vi "Shooter2 Controller.vi"(8 "error in":errorcluster) -> ()   [LabVIEW 2019]
doc: "This VI executes continuously carrying out the current operation and responding to updates or new operations. It will often contain the timing or control code that is difficult to place directly in TeleOp. This VI generally opens all sensors and motors and isolates the rest of the robot code from knowing how the operations are carried out."
uses:
  Shooter2 Setpoints.ctl
  Shooter2 Operations.ctl
  <vilib>/Rock Robotics/WPI/ThirdParty/Phoenix-LabVIEW/Motor Controller/Controls/CTRE_Phoenix_MotorControl_FeedbackDevice.ctl
  <vilib>/Rock Robotics/WPI/ThirdParty/Phoenix-LabVIEW/Motor Controller/Controls/CTRE_Phoenix_MotorControl_NeutralMode.ctl
  <vilib>/Rock Robotics/WPI/ThirdParty/Phoenix-LabVIEW/Motor Controller/Controls/CTRE_Phoenix_MotorControl_ControlMode.ctl
  <vilib>/Rock Robotics/WPI/ThirdParty/Phoenix-LabVIEW/Motor Controller/Get/CTRE_Phoenix_MotorController_GetSelectedSensorData.vi
  <vilib>/Rock Robotics/Network Tables/NT Write Boolean.vi
panel:
  out "Current\nCmd":string
  # "Tip: It may be helpful to observe inputs and sensor values.\nYou may also want to display tuning or debugging controls."
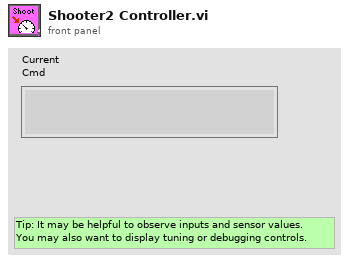
[diagram p1: front panel]
types:
  T1 = typedef "CTRE_Phoenix_MotorControl_ControlMode.ctl" = u16
  T2 = typedef "CTRE_Phoenix_MotorControl_NeutralMode.ctl" = enum8{"EEPROMSetting", "Override to Coast", "Override to Brake"}
  T3 = typedef "CTRE_Phoenix_MotorControl_FeedbackDevice.ctl" = i8
  T4 = typedef "Shooter2 Setpoints.ctl" = cluster{"Operation":T5, "Setpoint":dbl, "Duration":dbl}
  T5 = typedef "Shooter2 Operations.ctl" = enum16{"Reserve", "Read Current", "Immediate", "Shoot Manual", "Shoot Auto"}
  T6 = typedef "WPI_MotorControlDeviceRef.ctl" = cluster{"DeviceStatus":errorcluster, "Type":T7, "PWM":cluster{"PWM Channel":T8, "DeadBand":T9}, "CAN":cluster{"Device Number":u8, "SetOutput VI Ref":variant, "GetOutput VI Ref":variant, "Enable VI Ref":variant, "Disable VI Ref":variant, "Data":variant}, "Invert":bool, "DIO PWM":cluster{"PWM \"Enable\" Channel":T8, "DIOChannel":T10, "PWM Rate":dbl}}
  T7 = typedef "WPI_MotorControlType.ctl" = enum16{"PWM", "CAN", "DIO PWM"}
  T8 = typedef "FPGA_DIOPWMChannel.ctl" = enum8{"PWM 0", "PWM 1", "PWM 2", "PWM 3", "PWM 4", "PWM 5", "PWM 6", "PWM 7", "PWM 8", "PWM 9", "PWM MXP 0", "PWM MXP 1", "PWM MXP 2", "PWM MXP 3", "PWM MXP 4", "PWM MXP 5", "PWM MXP 6", "PWM MXP 7", "PWM MXP 8", "PWM MXP 9", "Invalid"}
  T9 = typedef "WPI_PWMDeadband.ctl" = cluster{"Name":string, "maxPositivePwm":i32, "minPositivePwm":i32, "centerPwm":i32, "maxNegativePwm":i32, "minNegativePwm":i32, "angularRange":u16}
  T10 = typedef "FPGA_DIOChannel.ctl" = enum8{"DIO 0", "DIO 1", "DIO 2", "DIO 3", "DIO 4", "DIO 5", "DIO 6", "DIO 7", "DIO 8", "DIO 9", "DIO MXP 0", "DIO MXP 1", "DIO MXP 2", "DIO MXP 3", "DIO MXP 4", "DIO MXP 5", "DIO MXP 6", "DIO MXP 7", "DIO MXP 8", "DIO MXP 9", "DIO MXP 10", "DIO MXP 11", "DIO MXP 12", "DIO MXP 13", "DIO MXP 14", "DIO MXP 15", "SPI Port CS1", "SPI Port CS2", "SPI Port CS3", "SPI Port MISO", "SPI Port MOSI", "Invalid"}
  T11 = typedef "Command Status Info.ctl" = cluster{"Name":string, "Status":T12, "notifier out":T13}
  T12 = typedef "Completion Status.ctl" = enum16{"Successful", "Aborted", "Incomplete"}
  T13 = typedef "Completion Notifier.ctl" = refnum<notifier>
  T14 = cluster{"Current Command":T4, "Command Timing":cluster{"Start Time (ms)":u32, "Iterations":i32}, "Command Arguments":cluster{"Command Info":T11, "Description":string, "Default Command":T4, "queue out":refnum<queue>, "Subsystem Name":string}}
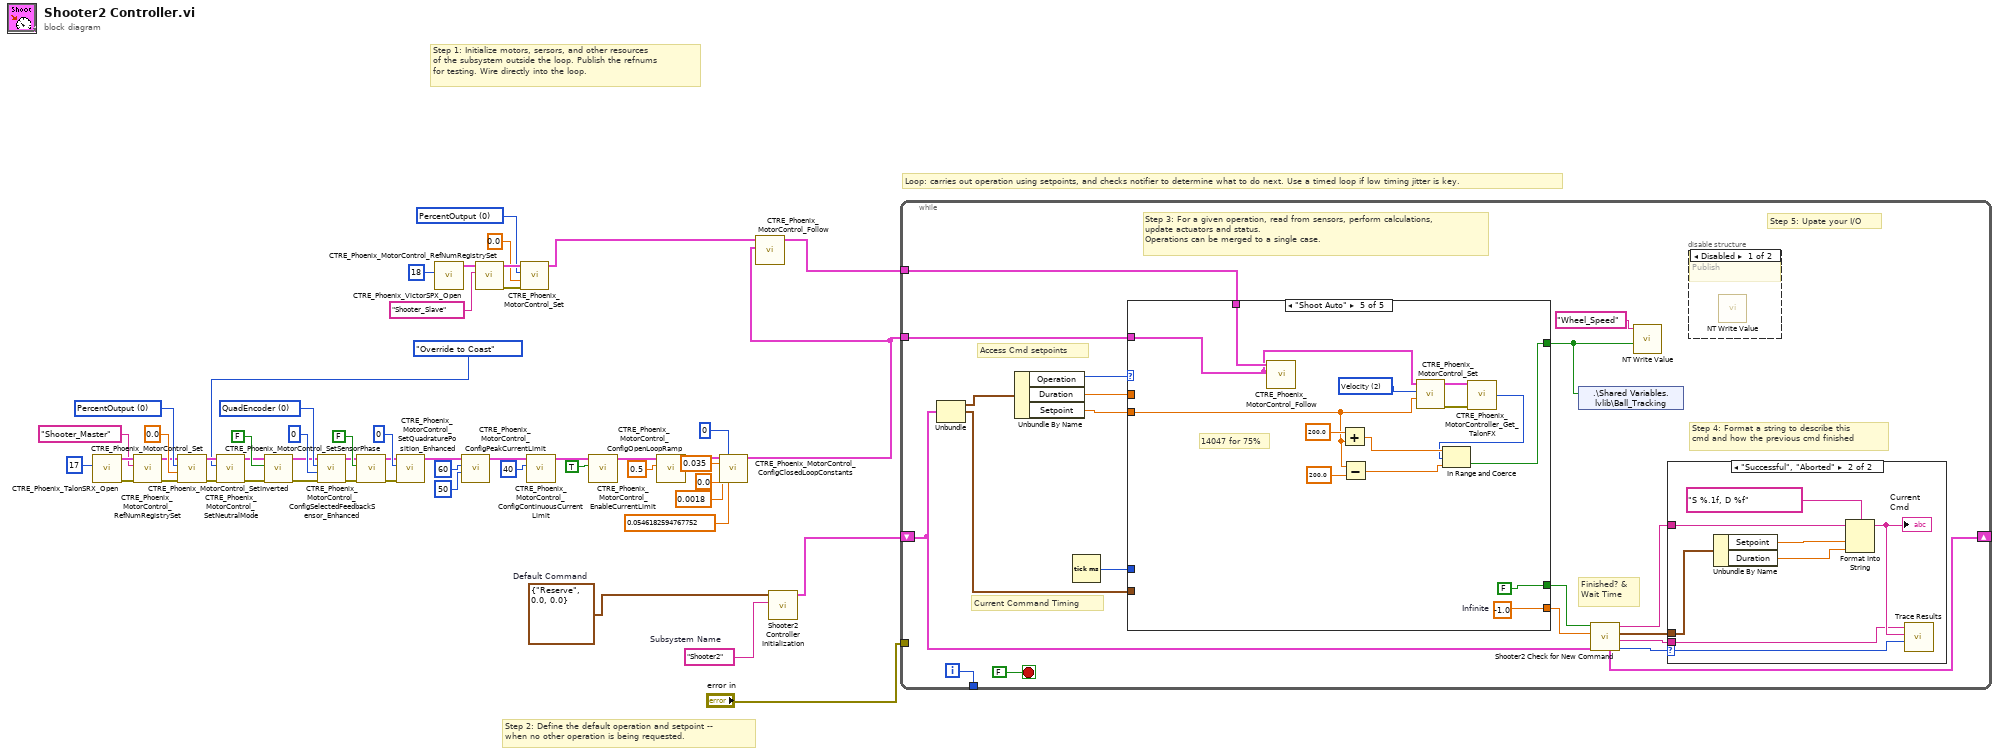
[diagram p0: block diagram]
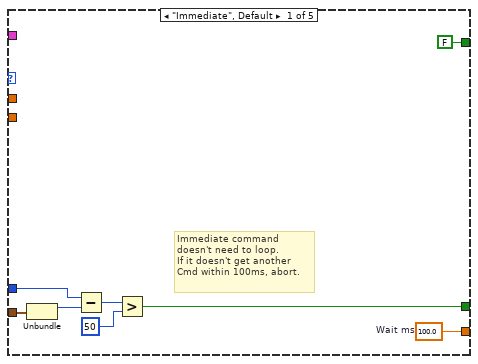
[diagram p4: hidden frame]
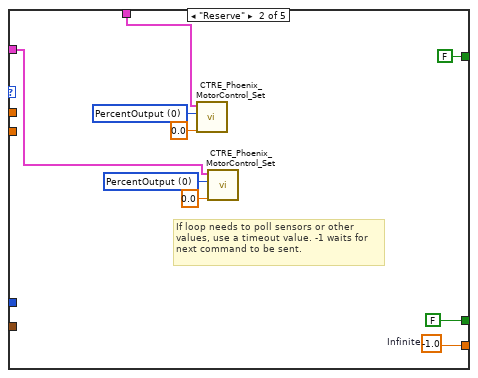
[diagram p5: hidden frame]
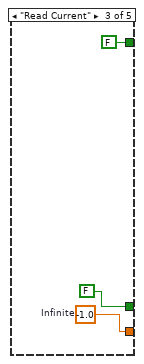
[diagram p6: hidden frame]
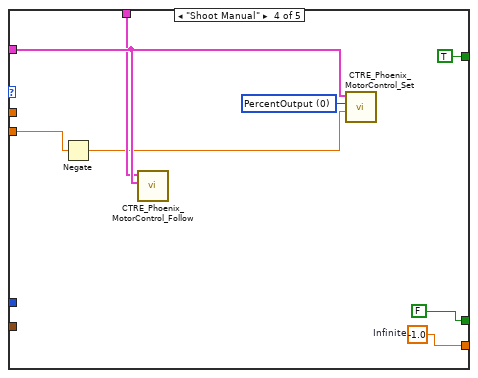
[diagram p7: hidden frame]
diagram:
  w19 = T1 0 items=["PercentOutput"=0, "Position"=1, "Velocity"=2, "Current"=3, "Follower"=5, "MotionProfile"=6, "MotionMagic"=7, "MotionProfileArc"=10, "Disabled"=15] ("Control Mode")
  w33 = T1 0 items=["PercentOutput"=0, "Position"=1, "Velocity"=2, "Current"=3, "Follower"=5, "MotionProfile"=6, "MotionMagic"=7, "MotionProfileArc"=10, "Disabled"=15] ("Control Mode")
  w46 = T3 0 items=["QuadEncoder"=0, "Analog"=2, "Tachometer"=4, "Pulse Width Encoded Position"=8, "Sensor Sum (S0 + S1)"=9, "Sensor Difference (D0 - D1)"=10, "Remote Source 0"=11, "Remote Source 1"=12, "Software Emulated"=15] ("Feedback Device")
  w49 = T4 {"Operation"=enum."Reserve", "Setpoint"=0.0, "Duration"=0.0}  # Default Command
  w50 = "Shooter2"  # Subsystem Name
  # "Step 2: Define the default operation and setpoint --\nwhen no other operation is being requested."
  # "Step 1: Initialize motors, sersors, and other resources\nof the subsystem outside the loop. Publish the refnums\nfor testing. Wire directly into the loop."
  # "Loop: carries out operation using setpoints, and checks notifier to determine what to do next. Use a timed loop if low timing jitter is key."
  n1 = call <vilib>:"CTRE_Phoenix_TalonSRX_Open.vi"("Device Number"=u8 17) -> ("error out"=w48:errorcluster, "CAN Talon SRX Ref"=w47:T6)  [unwired: 9 in]
  n2 = call <vilib>:"CTRE_Phoenix_MotorControl_RefNumRegistrySet.vi"("error in (no error)"=w48, "refnum name"="Shooter_Master", "PhoenixMotorControlDevRef"=w47) -> ("error out"=w30:errorcluster, "PhoenixMotorControlDevRef"=w31:T6)  [unwired: 7 in]
  n3 = call <vilib>:"CTRE_Phoenix_MotorControl_Set.vi"("error in (no error)"=w30, "Output"=0.0, "Control Mode"=w33, "PhoenixMotorControlDevRef"=w31) -> ("error out"=w29:errorcluster, "PhoenixMotorControlDevRef"=w35:T6)  [unwired: 6 in]
  n4 = call <vilib>:"CTRE_Phoenix_MotorControl_SetNeutralMode.vi"("error in (no error)"=w29, "Motor Control Neutral Mode"=CTRE_Phoenix_MotorControl_NeutralMode."Override to Coast", "PhoenixMotorControlDevRef"=w35) -> ("error out"=w28:errorcluster, "PhoenixMotorControlDevRef"=w36:T6)  [unwired: 7 in]
  n5 = call <vilib>:"CTRE_Phoenix_MotorControl_SetInverted.vi"("error in (no error)"=w28, "Invert?"=FALSE, "PhoenixMotorControlDevRef"=w36) -> ("error out"=w27:errorcluster, "PhoenixMotorControlDevRef"=w37:T6)  [unwired: 7 in]
  n6 = call <vilib>:"CTRE_Phoenix_MotorControl_ConfigSelectedFeedbackSensor_Enhanced.vi"("error in (no error)"=w27, "pidLoopIdx"=0, "Feedback Device"=w46, "PhoenixMotorControlDevRef"=w37) -> ("error out"=w39:errorcluster, "PhoenixMotorControlDevRef"=w41:T6)  [unwired: 6 in]
  n7 = call <vilib>:"CTRE_Phoenix_MotorControl_SetSensorPhase.vi"("error in (no error)"=w39, "PhaseSensor"=FALSE, "PhoenixMotorControlDevRef"=w41) -> ("error out"=w40:errorcluster, "PhoenixMotorControlDevRef"=w42:T6)  [unwired: 7 in]
  n8 = call <vilib>:"CTRE_Phoenix_MotorControl_SetQuadraturePosition_Enhanced.vi"("error in (no error)"=w40, "New Position"=0, "PhoenixMotorControlDevRef"=w42) -> ("PhoenixMotorControlDevRef"=w11:T6)  [unwired: 7 in, 1 out]
  n9 = call <vilib>:"CTRE_Phoenix_VictorSPX_Open.vi"("Device Number"=u8 18) -> ("CAN Talon SRX Ref"=w22:T6)  [unwired: 9 in, 1 out]
  n10 = call <vilib>:"CTRE_Phoenix_MotorControl_ConfigPeakCurrentLimit.vi"("Peak Current Maximum Duration (ms)"=50, "Peak Current (Amps)"=60, "PhoenixMotorControlDevRef"=w11) -> ("PhoenixMotorControlDevRef"=w13:T6)  [unwired: 7 in, 1 out]
  n11 = call <vilib>:"CTRE_Phoenix_MotorControl_RefNumRegistrySet.vi"("refnum name"="Shooter_Slave", "PhoenixMotorControlDevRef"=w22) -> ("error out"=w24:errorcluster, "PhoenixMotorControlDevRef"=w23:T6)  [unwired: 8 in]
  n12 = call <vilib>:"CTRE_Phoenix_MotorControl_Set.vi"("error in (no error)"=w24, "Output"=0.0, "Control Mode"=w19, "PhoenixMotorControlDevRef"=w23) -> ("PhoenixMotorControlDevRef"=w17:T6)  [unwired: 6 in, 1 out]
  n13 = call <vilib>:"CTRE_Phoenix_MotorControl_ConfigContinuousCurrentLimit.vi"("Continuous Current Limit (Amps)"=40, "PhoenixMotorControlDevRef"=w13) -> ("PhoenixMotorControlDevRef"=w12:T6)  [unwired: 8 in, 1 out]
  n14 = call <vilib>:"CTRE_Phoenix_MotorControl_EnableCurrentLimit.vi"("Enable Current Limit?"=TRUE, "PhoenixMotorControlDevRef"=w12) -> ("PhoenixMotorControlDevRef"=w8:T6)  [unwired: 8 in, 1 out]
  n15 = call <vilib>:"CTRE_Phoenix_MotorControl_ConfigOpenLoopRamp.vi"("secondsFromNeutralToFull"=0.5, "PhoenixMotorControlDevRef"=w8) -> ("PhoenixMotorControlDevRef"=w7:T6)  [unwired: 8 in, 1 out]
  n16 = call <vilib>:"CTRE_Phoenix_MotorControl_ConfigClosedLoopConstants.vi"("PhoenixMotorControlDevRef"=w7, "slotIdx"=0, "P"=0.035, "I"=0.0, "D"=0.0018, "F"=0.0546182594767752) -> ("PhoenixMotorControlDevRef"=w1:T6)  [unwired: 8 in, 1 out]
  n17 = call <vilib>:"CTRE_Phoenix_MotorControl_Follow.vi"("Master Controller to Follow"=w1, "PhoenixMotorControlDevRef"=w17) -> ()  [unwired: 8 in, 2 out]
  n18 = call "Shooter2 Controller Initialization.vi"("Subsystem Name"=w50, "Default Command"=w49) -> ("Current Command"=w51:T14)  [unwired: 9 in]
  n19 = while {
    shift-right: [w64] -> _
    shift-left: w51 -> [w57]
    tunnel: [w71] -> _
    tunnel: "error in" -> [_]
    tunnel: w1 -> [w56]
    tunnel: w17 -> [w55]
    i -> [w71]
    stop <- FALSE stop-if-true
    # "Step 5: Upate your I/O"
    # "Step 4: Format a string to describe this\ncmd and how the previous cmd finished"
    # "Current Command Timing"
    # "Access Cmd setpoints"
    # "Finished? &\nWait Time"
    # "Step 3: For a given operation, read from sensors, perform calculations,\nupdate actuators and status.\nOperations can be merged to a single case."
    n20 = Unbundle(w57) -> ("Current Command"=w70:T4, "Command Timing"=w66:cluster{"Start Time (ms)":u32, "Iterations":i32})  [unwired: 1 out]
    n21 = Unbundle By Name(w70) -> ("Operation"=w69:T5, "Duration"=w68:dbl, "Setpoint"=w65:dbl)
    n22 = Tick Count (ms)() -> (millisecond timer value=w67:u32)
    n23 = case shown="\"Shoot Auto\"" w69 {
      tunnel: [w88 w97 w99 w107 w122] -> w62
      tunnel: [w82 FALSE ("ignore previous (F)") FALSE ("ignore previous (F)") FALSE ("ignore previous (F)") FALSE ("ignore previous (F)")] -> w63
      tunnel: w66 -> [w84 _ _ _ _]
      tunnel: w68 -> [_ _ _ _ _]
      tunnel: w67 -> [w83 _ _ _ _]
      tunnel: w65 -> [_ _ _ w103 w111]
      tunnel: w56 -> [_ w91 _ w105 w118]
      tunnel: w55 -> [_ w90 _ w104 w119]
      tunnel: [FALSE FALSE FALSE TRUE w109] -> w53
      frame "Immediate", Default {
        w88 = 100.0  # Wait ms
        # "Immediate command\ndoesn't need to loop.\nIf it doesn't get another\nCmd within 100ms, abort."
        n24 = Unbundle(w84) -> ("Start Time (ms)"=w87:u32)  [unwired: 1 out]
        n25 = Subtract(x=w83, y=w87) -> (x-y=w86:u32)
        n26 = Greater?(x=w86, y=u8 50 ("Left Motor")) -> (0:w82:bool)
      }
      frame "Reserve" {
        w93 = T1 0 items=["PercentOutput"=0, "Position"=1, "Velocity"=2, "Current"=3, "Follower"=5, "MotionProfile"=6, "MotionMagic"=7, "MotionProfileArc"=10, "Disabled"=15] ("Control Mode")
        w95 = T1 0 items=["PercentOutput"=0, "Position"=1, "Velocity"=2, "Current"=3, "Follower"=5, "MotionProfile"=6, "MotionMagic"=7, "MotionProfileArc"=10, "Disabled"=15] ("Control Mode")
        w97 = -1.0  # Infinite
        # "If loop needs to poll sensors or other\nvalues, use a timeout value. -1 waits for\nnext command to be sent."
        n27 = call <vilib>:"CTRE_Phoenix_MotorControl_Set.vi"("Output"=0.0, "Control Mode"=w95, "PhoenixMotorControlDevRef"=w90) -> ()  [unwired: 7 in, 2 out]
        n28 = call <vilib>:"CTRE_Phoenix_MotorControl_Set.vi"("Output"=0.0, "Control Mode"=w93, "PhoenixMotorControlDevRef"=w91) -> ()  [unwired: 7 in, 2 out]
      }
      frame "Read Current" {
        w99 = -1.0  # Infinite
      }
      frame "Shoot Manual" {
        w106 = T1 0 items=["PercentOutput"=0, "Position"=1, "Velocity"=2, "Current"=3, "Follower"=5, "MotionProfile"=6, "MotionMagic"=7, "MotionProfileArc"=10, "Disabled"=15] ("Control Mode")
        w107 = -1.0  # Infinite
        n29 = Negate(x=w103) -> (-x=w102:dbl)
        n30 = call <vilib>:"CTRE_Phoenix_MotorControl_Follow.vi"("Master Controller to Follow"=w105, "PhoenixMotorControlDevRef"=w104) -> ()  [unwired: 8 in, 2 out]
        n31 = call <vilib>:"CTRE_Phoenix_MotorControl_Set.vi"("Output"=w102, "Control Mode"=w106, "PhoenixMotorControlDevRef"=w105) -> ()  [unwired: 7 in, 2 out]
      }
      frame "Shoot Auto" {
        w120 = T1 2 items=["PercentOutput"=0, "Position"=1, "Velocity"=2, "Current"=3, "Follower"=5, "MotionProfile"=6, "MotionMagic"=7, "MotionProfileArc"=10, "Disabled"=15] ("Control Mode")
        w122 = -1.0  # Infinite
        # "14047 for 75%"
        n32 = call <vilib>:"CTRE_Phoenix_MotorControl_Follow.vi"("Master Controller to Follow"=w118, "PhoenixMotorControlDevRef"=w119) -> ()  [unwired: 8 in, 2 out]
        n33 = Add(x=200.0, y=w111) -> (x+y=w114:dbl)
        n34 = Subtract(x=w111, y=200.0) -> (x-y=w115:dbl)
        n35 = call <vilib>:"CTRE_Phoenix_MotorControl_Set.vi"("Output"=w111, "Control Mode"=w120, "PhoenixMotorControlDevRef"=w118) -> ("error out"=w116:errorcluster, "PhoenixMotorControlDevRef"=w117:T6)  [unwired: 7 in]
        n36 = call-poly <vilib>:"CTRE_Phoenix_MotorController_Get_TalonFX.vi"("PhoenixMotorControlDevRef"=w117, "error in"=w116) -> ("Velocity (Raw Sensor Units per 100 ms)"=w110:i32)  [unwired: 10 in, 3 out]
        n37 = In Range and Coerce(upper limit=w114, x=w110, lower limit=w115) -> (In Range?=w109:bool)  [unwired: 1 out]
      }
    }
    n38 = shared-variable ".\\Shared Variables.lvlib\\Ball_Tracking"(w53) -> ()  [unwired: 1 in, 1 out]
    n39 = call "Shooter2 Check for New Command.vi"("Current Command"=w57, "Wait time (ms)"=w62, "Finished?"=w63) -> ("Completion"=w58:T12, "Subsystem Name"=w59:string, "Current Command"=w60:T4, "Initial Trace String"=w61:string, "NextCommand"=w64:T14)  [unwired: 4 in]
    n40 = call-poly <vilib>:"NT Write Value.vi"("Boolean"=w53, "Name"="Wheel_Speed") -> ()  [unwired: 9 in, 1 out]
    n41 = case shown="\"Successful\", \"Aborted\"" w58 {
      selector: w58 -> [_ w80]
      tunnel: w61 -> [_ w76]
      tunnel: w60 -> [_ w77]
      tunnel: w59 -> [_ w73]
      frame "Incomplete", Default {
        # "Continuing current command"
      }
      frame "Successful", "Aborted" {
        # "Report and setup for next command"
        n42 = Unbundle By Name(w77) -> ("Setpoint"=w79:dbl, "Duration"=w74:dbl)
        n43 = Format Into String(format string="S %.1f, D %f", initial string=w76, w79, w74) -> (resulting string=w75:string)  [unwired: 1 in, 1 out]
        "Current\nCmd" <- w75
        n44 = call <vilib>:"Trace Results.vi"("Status of previous command"=w80, "Description"=w75, "Subsystem"=w73) -> ()  [unwired: 9 in]
      }
    }
    n45 = disable-structure shown="Disabled" {
      frame Disabled {
        # "Publish"
        n46 = call-poly <vilib>:"NT Write Value.vi"() -> ()  [unwired: 11 in, 1 out]
      }
      frame Enabled {
      }
    }
  }
